vi "Measurement.UI.SetControllerDependency.vi"(8 "error in (no error)":errorcluster, 10 "Measurement":refnum<class "Measurement.lvclass">, 11 "Measurement.Free.UI in":refnum<class "Measurement.Free.UI.lvclass">) -> (0 "error out":errorcluster, 3 "Measurement.Free.UI out":refnum<class "Measurement.Free.UI.lvclass">)   [LabVIEW 2017, in "Measurement.Free.UI.lvclass"]
uses:
  Measurement.Free.UI.lvclass
  Measurement/Measurement.lvclass
  Measurement.Free/Measurement.Free.lvclass
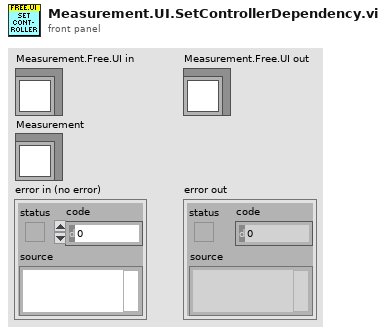
[diagram p1: front panel]
types:
  T1 = typedef "Measurement.Free.UI.lvclass/Dependencies--Cluster.ctl" = cluster{"Measurement.Free":refnum<class "Measurement.Free.lvclass">}
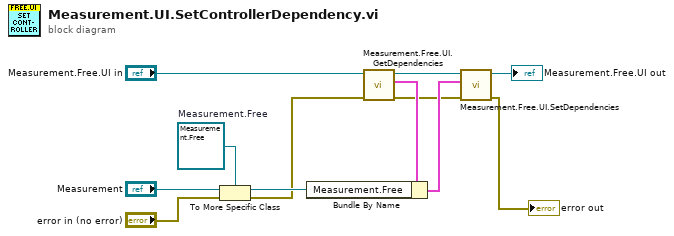
[diagram p0: block diagram]
diagram:
  w11 = refnum<class "Measurement.Free.lvclass"> refnum  # Measurement.Free
  n1 = To More Specific Class(target class=w11, reference="Measurement", error in="error in (no error)") -> (specific class reference=w7:refnum<class "Measurement.Free.lvclass">, error out=w3:errorcluster)
  n2 = call "Measurement.Free.UI.GetDependencies.vi"("error in (no error)"=w3, "Measurement.Free.UI in"="Measurement.Free.UI in") -> ("error out"=w2:errorcluster, "Dependencies"=w8:T1, "Measurement.Free.UI out"=w6:refnum<class "Measurement.Free.UI.lvclass">)  [unwired: 7 in]
  n3 = Bundle By Name(cluster=w8, "Measurement.Free"=w7) -> (w4:T1)
  n4 = call "Measurement.Free.UI.SetDependencies.vi"("error in (no error)"=w2, "Dependencies"=w4, "Measurement.Free.UI in"=w6) -> ("error out"=→"error out":errorcluster, "Measurement.Free.UI out"=→"Measurement.Free.UI out":refnum<class "Measurement.Free.UI.lvclass">)  [unwired: 7 in]
